vi "Generate Letters Coordinates.vi"() -> ()   [LabVIEW 2019, in "Display Utilities.lvlib"]
uses:
  Display Utilities.lvlib
  Display Element/Public/Controls/Vector.ctl
  Display Element/Display Element.lvclass
panel:
  out "Binary Image Inverted":bool[][](array[boolean])
  out "Coordenates":T1[](array[typedef])
  in  "Binary Image":bool[][](array[boolean])
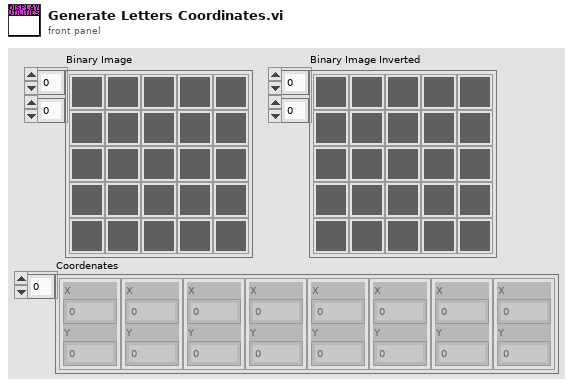
[diagram p1: front panel]
types:
  T1 = typedef "Display Element.lvclass/Vector.ctl" = cluster{"X":i32, "Y":i32}
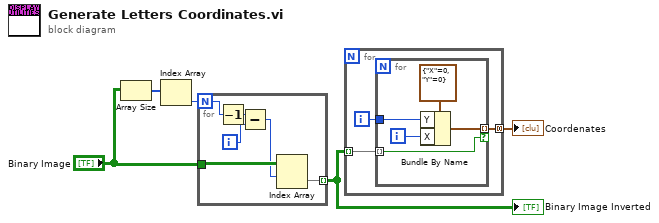
[diagram p0: block diagram]
diagram:
  n1 = Array Size(array="Binary Image") -> (size(s)=w2:i32[])
  n2 = Index Array(array=w2) -> (element=w1:i32)  [unwired: 1 in]
  n3 = for {
    N: w1 -> [w8]
    tunnel: "Binary Image" -> [w10]
    tunnel: [w6] -> w4 mode=indexing
    i -> [w11]
    n4 = Decrement(x=w8) -> (x-1=w7:i32)
    n5 = Subtract(x=w7, y=w11) -> (x-y=w9:i32)
    n6 = Index Array(array=w10, index (row)=w9) -> (element=w6:bool[])  [unwired: 1 in]
  }
  "Binary Image Inverted" <- w4
  n7 = for {
    tunnel: [w13] -> w5 mode=concatenating
    tunnel: w4 -> [w12] mode=indexing
    i -> [w14]
    n8 = for {
      tunnel: w14 -> [w18]
      tunnel: [w16] -> w13 mode=indexing if=w15
      tunnel: w12 -> [w15] mode=indexing
      i -> [w17]
      n9 = Bundle By Name(cluster=T1 {"X"=0, "Y"=0} ("Position"), "Y"=w18, "X"=w17) -> (w16:T1)
    }
  }
  "Coordenates" <- w5
